vi "Send Message.vi"(7 "Data DVR":refnum<data-value>, 8 "error in (no error)":errorcluster, 11 "Message Type in":refnum<class "Communication.lvclass">) -> (0 "error out":errorcluster, 3 "Message Type out":refnum<class "Communication.lvclass">)   [LabVIEW 2023, in "Communication.lvclass"]
uses:
  Communication.lvclass
  Data/Data.lvclass
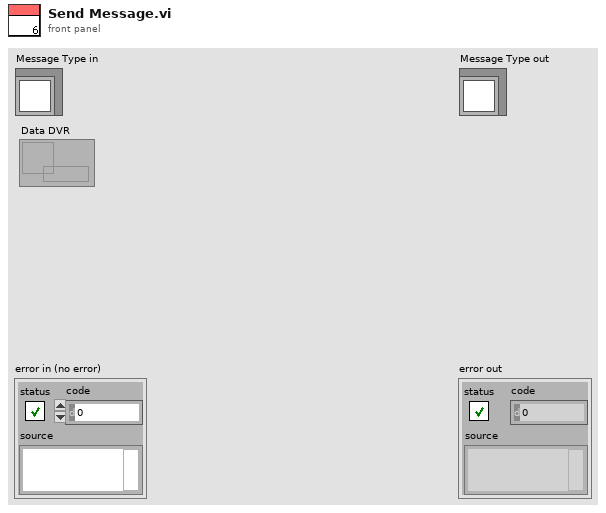
[diagram p1: front panel]
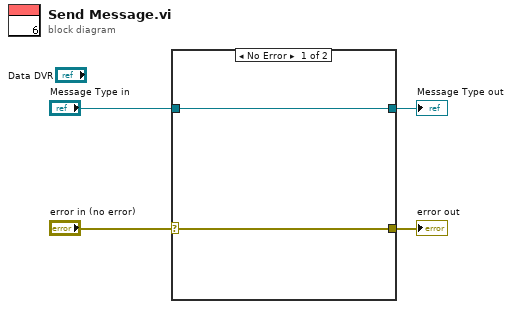
[diagram p0: block diagram]
diagram:
  n1 = case shown="No Error" "error in (no error)" {
    selector: "error in (no error)" -> [w5 w8]
    tunnel: [w5 w8] -> w3
    tunnel: [w6 w7] -> w1
    tunnel: "Message Type in" -> [w6 w7]
    frame No Error {
    }
    frame Error {
    }
  }
  "error out" <- w3
  "Message Type out" <- w1
